vi "Measure Harmonic Distortion.vi"(9 "Auto cal (F)?":bool, 11 "State":T1) -> (0 "error out":errorcluster)   [LabVIEW 2015]
uses:
  Utility VIs/Type Defs/Speaker ring.ctl
  Utility VIs/Buttons/KCheckmarkBoolean 2.ctl
  Cochlear Function Test Suite/LV Source/CFTS Main Panel SubVIs/CFTS-Experiment State.ctl
  Type Defs/ACal-In Ear Parameters.ctl
  Type Defs/Cal Stimulus.ctl
  Type Defs/ACal-Multiband Parameters.ctl
  Utility VIs/Conversion VIs/Create Waveform Cluster (2D).vi
  Utility VIs/Math VIs/FFT x(t) to dB,Degrees (2D).vi
  Instance           1 24Saved   Calibrate In Ear .vi
  Utility VIs/File IO VIs/Configuration File Wrapper VIs/Config-Read Key (Boolean).vi
panel:
  in  "Weighted":bool
  out "Auto Message":string="Auto calibrating!"
  in  "Speaker":T2
  in  "mic gain":dbl caption="Probe Mic Gain (dB)"
  in  "Stimulus":T3={"Min Freq (Hz)"=1000.0, "Max Freq (Hz)"=50000.0, "Freq Step (Hz)"=50.0, "Waveform"=0, "Attenuation (dB)"=30.0, "Sample Rate (Hz)"=100000.0} {"Waveform" items=["Chirp", "Weighted"]}
  out "Stimulus graph":cluster{i32, dbl, dbl[]}(graph)={0, 0.01, []}
  in  "Averages":i32=128
  in  "Return":bool
  in  "START":bool
  in  "STOP":bool
  in  "result":cluster{"Path":path, "error ":errorcluster}
  in  "Plot Max SPL":T4=TRUE
  out "ASTF":cluster{"Frequency":dbl[], "Frequency":dbl[]}[](graph)
  in  "Last N":bool
  in  "Show all":bool
  in  "Load":bool
  in  "Clear":bool
  out "Path":path
  out "Acquired":i32=256
  out "ASTF phase":cluster{"Frequency":dbl[], "Frequency":dbl[]}[](graph)
  out "Mic phase graph":cluster{"offset":dbl, "dx":dbl, "Y":dbl[][]}(graph)
  out "Mic mag":cluster{"offset":dbl, "dx":dbl, "Y":dbl[][]}(graph)
  out "Mic signals":cluster{"offset":dbl, "dx":dbl, "Y":dbl[][]}(graph)
  # "Raw Data"
  # "Acoustic System Transfer Function"
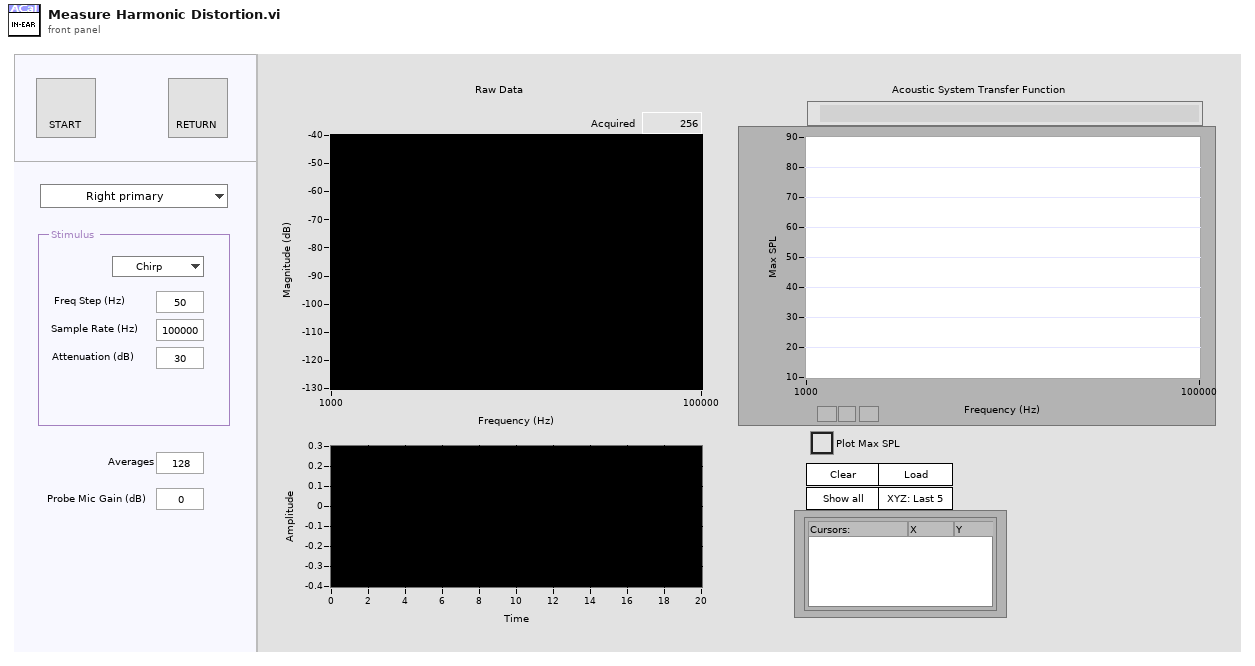
[diagram p1: front panel]
types:
  T1 = typedef "CFTS-Experiment State.ctl" = cluster{"Experimenter":string, "Number":u32, "Right":string, "Left":string, "Data Folder":path, "State File":path, "Version Info":string, "End Exposure Time":dbl, "Exposure Duration":string, "Run #":cluster{"CAP":i16, "ABR":i16, "DP":i16, "VsEP":i16, "MeasSeq":i16, "SubSeq":i16, "SFOAE":i16}}
  T2 = typedef "Speaker ring.ctl" = enum16{"Right primary", "Right secondary", "Left primary", "Left secondary"}
  T3 = cluster{"Min Freq (Hz)":dbl, "Max Freq (Hz)":dbl, "Freq Step (Hz)":dbl, "Waveform":u16, "Attenuation (dB)":dbl, "Sample Rate (Hz)":dbl}
  T4 = typedef "KCheckmarkBoolean 2.ctl" = bool
  T5 = typedef "ACal-In Ear Parameters.ctl" = cluster{"Speaker":T2, "Stimulus":T6, "Averages":i32, "Left gain":dbl, "Right gain":dbl, "plot max":bool, "smooth override":bool, "Weighted":T7}
  T6 = typedef "Cal Stimulus.ctl" = cluster{"Min Freq (Hz)":dbl, "Max Freq (Hz)":dbl, "Freq Step (Hz)":dbl, "Waveform":enum16{"Chirp", "Weighted"}, "Attenuation (dB)":dbl, "Sample Rate (Hz)":dbl}
  T7 = typedef "ACal-Multiband Parameters.ctl" = cluster{"Folder":path, "Fmin":dbl, "Fmax":dbl, "Max range":dbl, "WF":u16}
  T8 = typedef "Cal-Smoothing Parameters.ctl" = cluster{"Method":enum16{"None", "Moving average", "Loess"}, "MA":cluster{"Iterations":i32, "Length":i32}, "Loess":cluster{"Length":i32, "Type":enum16{"Linear", "Quadratic"}, "Robust":bool}}
  T9 = cluster{"new file path":path, "error out":errorcluster}
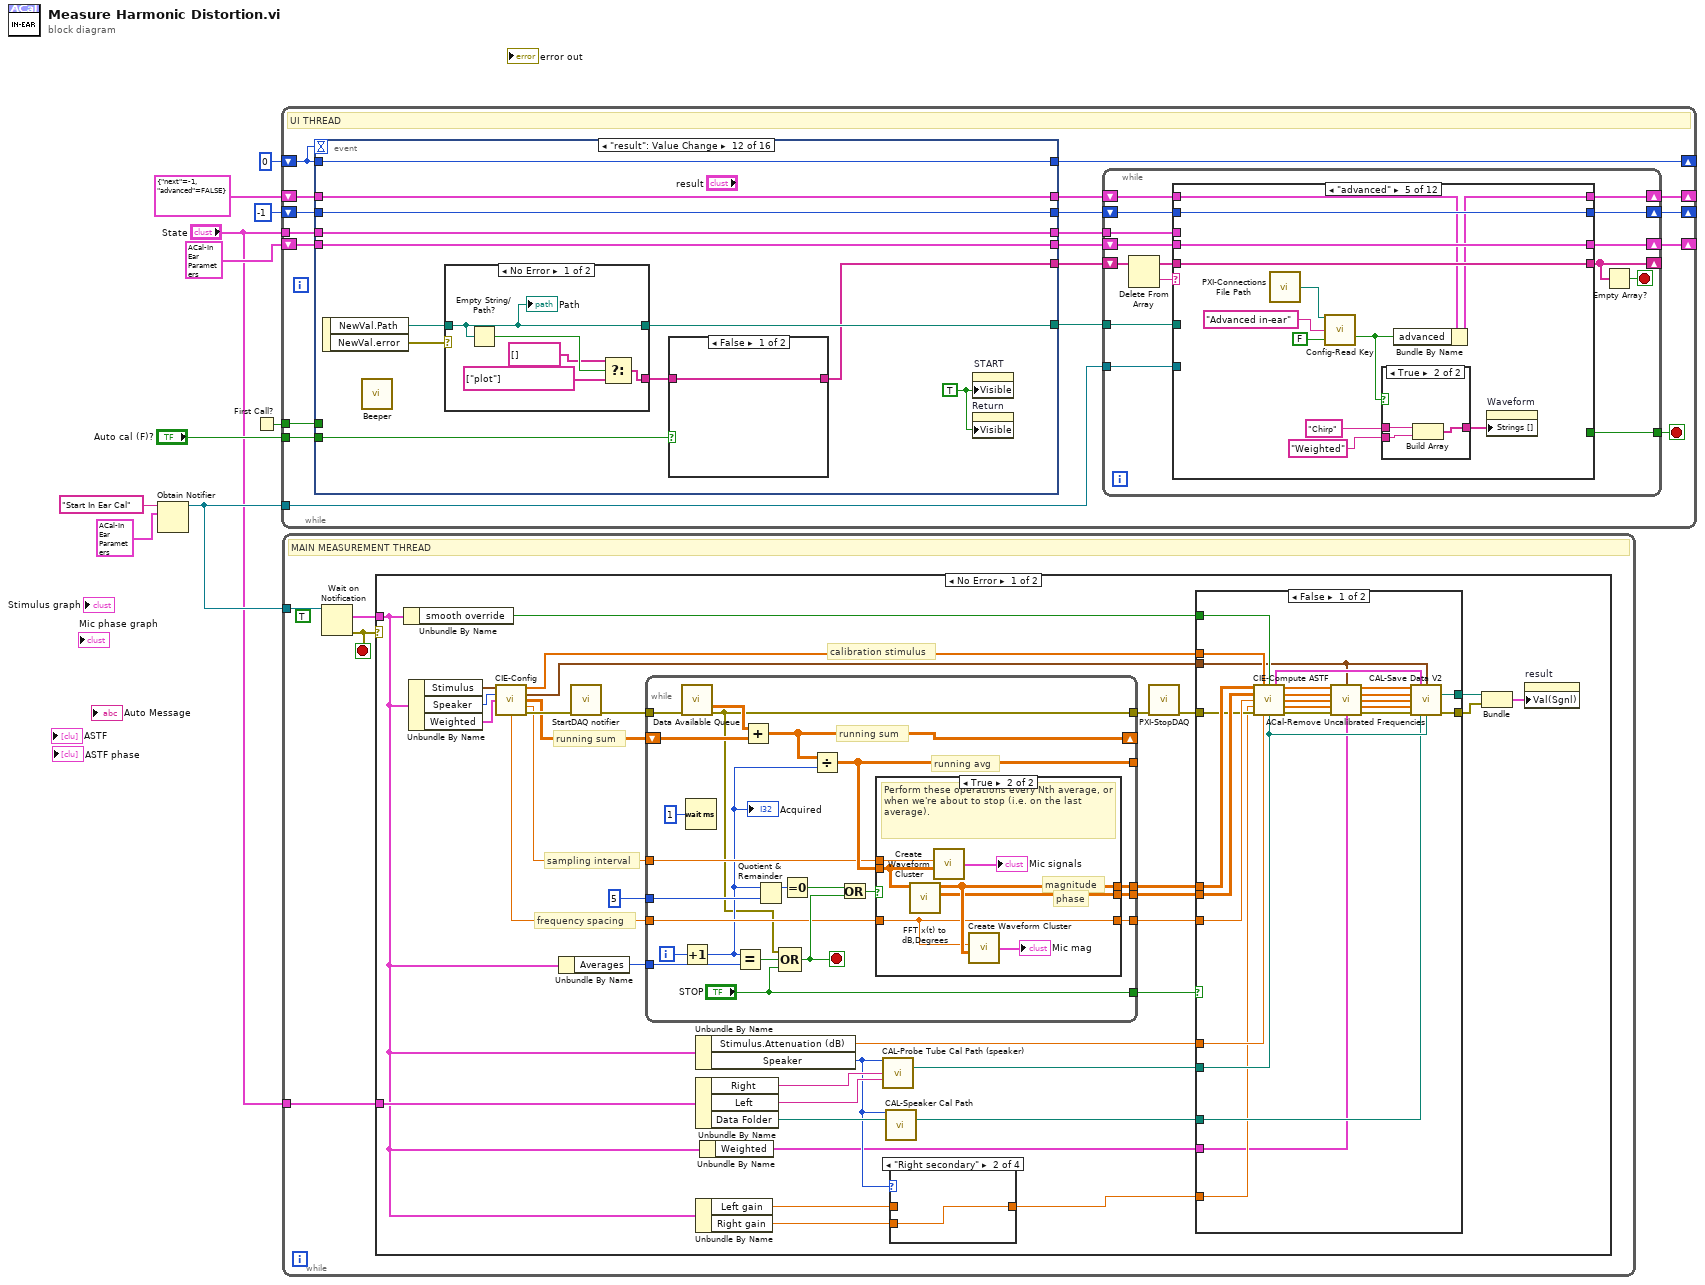
[diagram p0: block diagram]
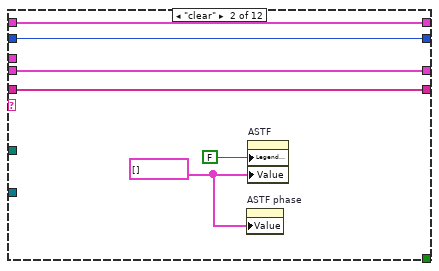
[diagram p9: hidden frame]
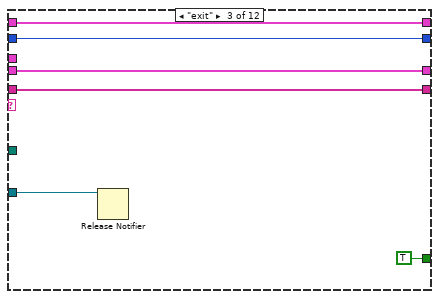
[diagram p10: hidden frame]
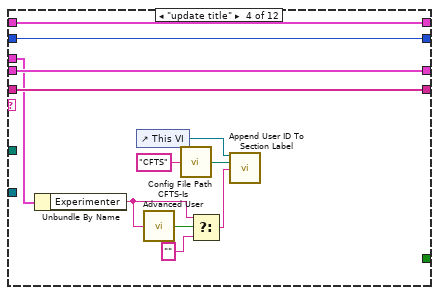
[diagram p11: hidden frame]
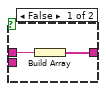
[diagram p12: hidden frame]
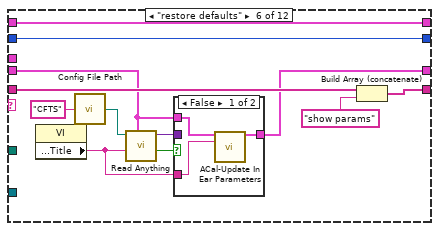
[diagram p13: hidden frame]
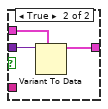
[diagram p14: hidden frame]
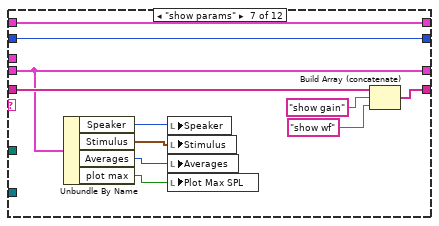
[diagram p15: hidden frame]
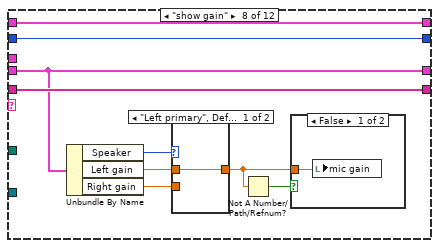
[diagram p16: hidden frame]
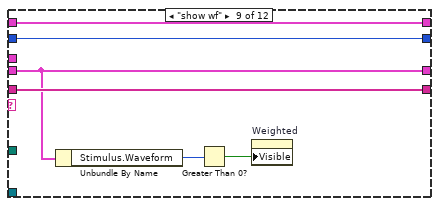
[diagram p19: hidden frame]
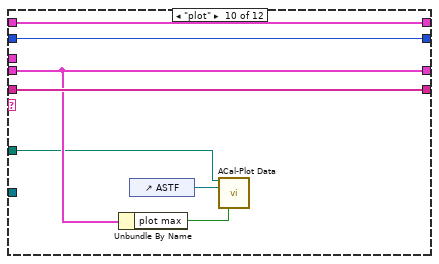
[diagram p20: hidden frame]
diagram:
  n1 = Obtain Notifier(name (unnamed)="Start In Ear Cal", notification data type=T5 {"Speaker"=enum."Right primary", "Stimulus"={"Min Freq (Hz)"=50.0, "Max Freq (Hz)"=50000.0, "Freq Step (Hz)"=50.0, "Waveform"=enum."Chirp", "Attenuation (dB)"=20.0, "Sample Rate (Hz)"=100000.0}, "Averages"=512, "Left gain"=40.0, "Right gain"=40.0, "plot max"=TRUE, "smooth override"=FALSE, "Weighted"={"Folder"=path "", "Fmin"=0.0, "Fmax"=0.0, "Max range"=0.0, "WF"=0}} ("Params")) -> (notifier out=w10:refnum<notifier>)  [unwired: 2 in, 2 out]
  n2 = First Call?() -> (First Call?: T/F=w1:bool)
  n3 = while {
    tunnel: w10 -> [w17]
    shift-right: [w26] -> _
    shift-left: 0 -> [w27]
    tunnel: "Auto cal (F)?" -> [w29]
    shift-right: [w20] -> _
    shift-left: -1 -> [w28]
    tunnel: "State" -> [w25]
    shift-right: [w21] -> _
    shift-left: T5 {"Speaker"=enum."Right primary", "Stimulus"={"Min Freq (Hz)"=50.0, "Max Freq (Hz)"=50000.0, "Freq Step (Hz)"=50.0, "Waveform"=enum."Chirp", "Attenuation (dB)"=20.0, "Sample Rate (Hz)"=100000.0}, "Averages"=512, "Left gain"=40.0, "Right gain"=40.0, "plot max"=TRUE, "smooth override"=FALSE, "Weighted"={"Folder"=path "C:/Data", "Fmin"=3000.0, "Fmax"=45000.0, "Max range"=25.0, "WF"=0}} ("Params") -> [w24]
    shift-right: [w12] -> _
    shift-left: cluster{"next":i32, "advanced":bool} {"next"=-1, "advanced"=FALSE} -> [w14]
    tunnel: w1 -> [w11]
    stop <- w18 stop-if-true
    # "UI THREAD"
    n4 = event shown="[11] \"result\": Value Change" {
      selector: _ -> [_ _ _ _ _ _ _ _ _ _ _ _ _ _ _ _]
      dyn-events: _ -> [_ _ _ _ _ _ _ _ _ _ _ _ _ _ _ _]
      timeout: w27 -> [_ _ _ _ _ _ _ _ _ _ _ _ _ _ _ _]
      tunnel: w29 -> [w184 _ _ _ _ _ _ _ _ _ _ w307 _ _ _ _]
      tunnel: w28 -> [w185 w202 w211 w233 w239 w247 w250 w263 w265 w278 w291 w315 w331 w338 w353 w363]
      tunnel: [w185 w202 w211 w233 w239 w247 w250 w263 w265 w278 w291 w315 w331 w338 w353 w363] -> w23
      tunnel: w27 -> [_ w201 w210 w232 w238 w246 w255 w262 w270 w277 w290 w314 w330 w337 w351 w361]
      tunnel: [-1 w201 w210 w232 w238 w246 w255 w262 w270 w277 w290 w314 w330 w337 w351 w361] -> w26
      tunnel: w25 -> [w180 w198 w205 w229 w237 w241 w253 w261 w268 w273 w288 w312 w327 w335 w350 w360]
      tunnel: w24 -> [w182 w200 w208 w231 w236 w245 w254 w259 w269 w275 w289 w313 w329 w336 w349 w359]
      tunnel: [w182 w200 w207 w231 w236 w243 w252 w257 w267 w274 w287 w313 w329 w336 w349 w359] -> w22
      tunnel: [w179 string[] ["exit"] w206 string[] ["exit"] string[] ["start"] string[] ["show gain"] string[] ["show wf"] _ _ _ _ w305 string[] ["clear"] w333 _ _] -> w19
      tunnel: [w180 w198 w205 w229 w237 w241 w253 w261 w268 w273 w288 w312 w327 w335 w350 w360] -> w16
      tunnel: [_ _ _ _ _ _ _ _ _ _ _ w310 _ w334 _ _] -> w15
      tunnel: w14 -> [w177 w197 w204 w228 w235 w240 w249 w260 w264 w271 w285 w309 w326 w332 w347 w356]
      tunnel: [w177 w197 w204 w228 w235 w240 w249 w260 w264 w271 w285 w309 w326 w332 w347 w356] -> w13
      tunnel: w11 -> [w175 _ _ _ _ _ _ _ _ _ _ _ _ _ _ _]
      event Timeout {
        w191 = TRUE ("Visible")
        n5 = event-data() -> ()  [unwired: 1 in, 1 out]
        n6 = case shown="False" w184 {
          tunnel: [w193 string[] ["next", "clear"]] -> w181
          tunnel: w175 -> [w195 _]
          frame False {
            n7 = Select(t=string[] ["clear"], s=w195, f=string[] []) -> (s? t:f=w193:string[])
          }
          frame True {
          }
        }
        n8 = property on="Auto Message" class="Str"("Visible"=w184, "Blinking"=w184) -> ()  [unwired: 2 in, 2 out]
        n9 = Unbundle By Name(w180) -> ("Experimenter"=w190:string)
        n10 = property on="Weighted" class="Bool"("Visible"=FALSE) -> ()  [unwired: 2 in, 2 out]
        n11 = Concatenate Strings(w190, ": Last 5" ("string")) -> (w188:string)
        n12 = property on="START" class="Bool"("Visible"=w191) -> ()  [unwired: 2 in, 2 out]
        n13 = property on="Return" class="Bool"("Visible"=w191) -> ()  [unwired: 2 in, 2 out]
        n14 = Initialize Array(w188, 4 ("dimension size")) -> (w186:string[])
        n15 = property on="Last N" class="Bool"("Strings [4]"=w186) -> ()  [unwired: 2 in, 2 out]
        n16 = Build Array (concatenate)(w181, string[] ["restore defaults", "advanced", "update title"]) -> (w179:string[])
      }
      event Panel Close? {
        n17 = event-data() -> ()  [unwired: 1 in, 1 out]
        n18 = event-data("Discard?"=TRUE) -> ()  [unwired: 1 in, 1 out]
      }
      event Menu Selection (User) {
        n19 = event-data() -> ("ItemTag"=w209:string)  [unwired: 1 in]
        n20 = case shown="\"mmFileSave\"" w209 {
          tunnel: w208 -> [w212 w214 w217 w223 w226]
          tunnel: [w212 w214 w217 w223 w224] -> w207
          tunnel: [_ string[] ["restore defaults"] _ string[] ["exit"] _] -> w206
          frame "", Default {
          }
          frame "mmFileRestore" {
          }
          frame "mmFileSave" {
            n21 = property class="VI"() -> ("Front Panel.Title"=w216:string)  [unwired: 2 in, 2 out]
            n22 = call "Config File Path.vi"("AppName"="CFTS") -> ("Default config file name"=w218:path)
            n23 = call "Write Anything.vi"("Section Name (Name of \"Anything\")"=w216, "Anything"=w217, "Path (dialog)"=w218) -> ("Error Out"=w215:errorcluster)  [unwired: 7 in, 1 out]
            n24 = case shown="Error" w215 {
              selector: w215 -> [_ w221]
              frame No Error {
                n25 = One Button Dialog(message="Defaults saved.") -> ()  [unwired: 1 in, 1 out]
              }
              frame Error {
                n26 = call "Error Handler.vi"("error in (no error)"=w221) -> ()  [unwired: 13 in, 2 out]
              }
            }
          }
          frame "mmFileExit" {
          }
          frame "mmEditOptions" {
            n27 = Unbundle By Name(w226) -> ("smooth override"=w227:bool)
            n28 = call "CIE-Options Dialog.vi"("Override smoothing"=w227) -> ("Override Out"=w225:bool)  [unwired: 13 in, 1 out]
            n29 = Bundle By Name(cluster=w226, "smooth override"=w225) -> (w224:T5)
          }
        }
      }
      event "Return": Value Change {
        n30 = event-data() -> ()  [unwired: 1 in, 1 out]
      }
      event "START": Value Change {
        n31 = event-data() -> ()  [unwired: 1 in, 1 out]
      }
      event Value Change {
        n32 = event-data() -> ("NewVal"=w242:T2)  [unwired: 1 in]
        n33 = Bundle By Name(cluster=w245, "Speaker"=w242) -> (w243:T5)
      }
      event "Stimulus": Value Change {
        n34 = event-data() -> ()  [unwired: 1 in, 1 out]
        n35 = Bundle By Name(cluster=w254, "Stimulus"="Stimulus") -> (w252:T5)
      }
      event "Weighted": Value Change {
        n36 = event-data() -> ()  [unwired: 1 in, 1 out]
        n37 = Unbundle By Name(w259) -> ("Weighted"=w258:T7)
        n38 = call "ACal-Multiband Dialog.vi"("Cluster In"=w258) -> ("Cluster out"=w256:T7)  [unwired: 13 in, 1 out]
        n39 = Bundle By Name(cluster=w259, "Weighted"=w256) -> (w257:T5)
      }
      event "Averages": Value Change {
        n40 = event-data() -> ()  [unwired: 1 in, 1 out]
        n41 = Bundle By Name(cluster=w269, "Averages"="Averages") -> (w267:T5)
      }
      event "mic gain": Value Change {
        n42 = event-data() -> ()  [unwired: 1 in, 1 out]
        n43 = Unbundle By Name(w275) -> ("Speaker"=w276:T2)
        n44 = case shown="\"Right primary\", \"Right secondary\"" w276 {
          tunnel: w275 -> [w281 w284]
          tunnel: [w280 w283] -> w274
          tunnel: "mic gain" -> [w279 w282]
          frame "Left primary", Default {
            n45 = Bundle By Name(cluster=w281, "Left gain"=w279) -> (w280:T5)
          }
          frame "Right primary", "Right secondary" {
            n46 = Bundle By Name(cluster=w284, "Right gain"=w282) -> (w283:T5)
          }
        }
      }
      event Value Change {
        # "Clear the plot because the scaling is no longer consistent with the option. We haven't retained a list of displayed data files, so we can't restore them with the proper scaling. The best we can do (without more serious revision) is to reload the last saved calibration file."
        n47 = event-data() -> ("NewVal"=w296:T4)  [unwired: 1 in]
        n48 = control-ref of="ASTF"() -> (w294:refnum<vi>)
        n49 = property class="XYGraph (strict)"(reference=w294, "Value"=cluster{"Frequency":dbl[], "Frequency":dbl[]}[] []) -> (reference out=w292:refnum<vi>, error out=w295:errorcluster)  [unwired: 1 in]
        n50 = Bundle By Name(cluster=w289, "plot max"="Plot Max SPL") -> (w287:T5)
        n51 = local read "Path"() -> (w298:path)
        n52 = call "FileIO-File or Folder Exists.vi"("error in (no error)"=w295, "path"=w298) -> ("Directory?"=w299:bool, "dup path"=w297:path)  [unwired: 6 in, 2 out]
        n53 = case shown="True" w299 {
          tunnel: w292 -> [_ w302]
          tunnel: w296 -> [_ w300]
          tunnel: w297 -> [_ w303]
          frame False {
          }
          frame True {
            n54 = call "ACal-Plot Data.vi"("Path"=w303, "Mag graph"=w302, "Plot max"=w300) -> ("error out"=w301:errorcluster)  [unwired: 11 in, 1 out]
            n55 = call <vilib>:"Simple Error Handler.vi"("error in (no error)"=w301) -> ()  [unwired: 4 in, 5 out]
          }
        }
      }
      event "result": Value Change {
        w308 = TRUE
        n56 = event-data() -> ("NewVal.Path"=w311:path, "NewVal.error"=w304:errorcluster)  [unwired: 1 in]
        n57 = call "Beeper.vi"() -> ()  [unwired: 5 in, 1 out]
        n58 = case shown="No Error" w304 {
          selector: w304 -> [_ w325]
          tunnel: w311 -> [w324 _]
          tunnel: [w324 _] -> w310
          tunnel: [w321 _] -> w306
          frame No Error {
            n59 = Empty String/Path?(string/path=w324) -> (empty?=w323:bool)
            n60 = Select(t=string[] [], s=w323, f=string[] ["plot"]) -> (s? t:f=w321:string[])
            "Path" <- w324
          }
          frame Error {
            n61 = call "Error Handler.vi"("error in (no error)"=w325) -> ()  [unwired: 13 in, 2 out]
          }
        }
        n62 = case shown="False" w307 {
          tunnel: w306 -> [w316 w319]
          tunnel: [w316 w318] -> w305
          frame False {
          }
          frame True {
            n63 = Build Array (concatenate)("next", w319) -> (w318:string[])
          }
        }
        n64 = property on="START" class="Bool"("Visible"=w308) -> ()  [unwired: 2 in, 2 out]
        n65 = property on="Return" class="Bool"("Visible"=w308) -> ()  [unwired: 2 in, 2 out]
      }
      event "Clear": Value Change {
        n66 = event-data() -> ()  [unwired: 1 in, 1 out]
      }
      event "Load": Value Change {
        n67 = event-data() -> ()  [unwired: 1 in, 1 out]
        n68 = Unbundle By Name(w335) -> ("Data Folder"=w339:path)
        n69 = call "File Dialog"("start path"=w339, "pattern (all files)"="*.calib", "pattern label"="Calibration files") -> ("selected path"=w344:path, "cancelled"=w343:bool, "error out"=w342:errorcluster)  [unwired: 9 in, 1 out]
        n70 = case shown="False" w343 {
          tunnel: w344 -> [w346 _]
          tunnel: w342 -> [_ _]
          tunnel: [w346 _] -> w334
          tunnel: [string[] ["plot"] _] -> w333
          frame False {
          }
          frame True {
          }
        }
      }
      event "Show all": Value Change {
        n71 = event-data() -> ()  [unwired: 1 in, 1 out]
        n72 = Unbundle By Name(w349) -> ("plot max"=w348:bool)
        n73 = Unbundle By Name(w350) -> ("Data Folder"=w354:path)
        n74 = control-ref of="ASTF"() -> (w352:refnum<vi>)
        n75 = call "CAL-Show all.vi"("Path"=w354, "Mag graph"=w352, "Plot Max SPL"=w348) -> ("error out"=w355:errorcluster)  [unwired: 11 in, 1 out]
        n76 = call "Error Handler.vi"("error in (no error)"=w355) -> ()  [unwired: 13 in, 2 out]
      }
      event "Last N": Value Change {
        n77 = event-data() -> ()  [unwired: 1 in, 1 out]
        n78 = Unbundle By Name(w359) -> ("Speaker"=w357:T2, "plot max"=w358:bool)
        n79 = control-ref of="ASTF"() -> (w362:refnum<vi>)
        n80 = call "CAL-Show Last N.vi"("Expt State"=w360, "Mag graph"=w362, "Speaker"=w357, "Plot Max SPL"=w358) -> ("error out"=w364:errorcluster)  [unwired: 11 in]
        n81 = call <vilib>:"Simple Error Handler.vi"("error in (no error)"=w364) -> ()  [unwired: 4 in, 5 out]
      }
    }
    n82 = while {
      shift-right: [w42] -> w21
      shift-left: w22 -> [w43]
      shift-right: [w41] -> w20
      shift-left: w23 -> [w44]
      shift-right: [w37] -> _
      shift-left: w19 -> [w39]
      tunnel: w17 -> [w35]
      tunnel: [w34] -> w18
      tunnel: w16 -> [w33]
      tunnel: w15 -> [w32]
      shift-right: [w31] -> w12
      shift-left: w13 -> [w30]
      stop <- w36 stop-if-true
      n83 = Delete From Array(array=w39) -> (deleted portion=w38:string, array with subset deleted=w40:string[])  [unwired: 2 in]
      n84 = case shown="\"advanced\"" w38 {
        tunnel: w44 -> [w48 w54 w60 w72 w84 w101 w118 w127 w136 w143 w149 w162]
        tunnel: [w48 w54 w60 w72 w84 w101 w118 w127 w136 w143 w149 w162] -> w41
        tunnel: w43 -> [w47 w53 w59 w71 w83 w96 w116 w125 w133 w141 w144 w155]
        tunnel: [w47 w53 w59 w71 w83 w95 w116 w125 w133 w141 w144 w154] -> w42
        tunnel: w40 -> [w46 w52 w58 w70 w82 w100 w117 w126 w135 w142 w145 w153]
        tunnel: [w46 w52 w58 w70 w82 w94 w111 w126 w135 w142 w145 w150] -> w37
        tunnel: w35 -> [_ _ w57 _ _ _ _ _ _ _ w146 _]
        tunnel: [_ _ TRUE _ _ _ _ _ _ _ _ w158] -> w34
        tunnel: w33 -> [_ _ _ w63 _ _ _ _ _ _ _ _]
        tunnel: w32 -> [_ _ _ _ _ _ _ _ _ w138 _ _]
        tunnel: [w45 w49 w55 w61 w77 w90 w109 w119 w134 w137 w148 w151] -> w31
        tunnel: w30 -> [w45 w49 w55 w61 w78 w90 w109 w119 w134 w137 w148 w152]
        frame "", Default {
        }
        frame "clear" {
          w51 = cluster{"Frequency":dbl[], "Frequency":dbl[]}[] [] ("ASTF mag")
          n85 = property on="ASTF phase" class="XYGraph (strict)"("Value"=w51) -> ()  [unwired: 2 in, 2 out]
          n86 = property on="ASTF" class="XYGraph (strict)"("Legend Visible"=FALSE ("Legend:Visible"), "Value"=w51) -> ()  [unwired: 2 in, 2 out]
        }
        frame "exit" {
          n87 = Release Notifier(notifier=w57) -> ()  [unwired: 2 in, 3 out]
        }
        frame "update title" {
          n88 = Unbundle By Name(w63) -> ("Experimenter"=w62:string)
          n89 = control-ref of="This VI"() -> (w64:refnum<vi>)
          n90 = call "CFTS-Is Advanced User.vi"("Experimenter"=w62) -> ("Advanced user"=w67:bool)
          n91 = call "Config File Path.vi"("AppName"="CFTS") -> ("Default config file name"=w65:path)
          n92 = Select(t=w62, s=w67, f="") -> (s? t:f=w69:string)
          n93 = call "Append User ID To Section Label.vi"("VI reference"=w64, "Path (dialog)"=w65, "User"=w69) -> ()  [unwired: 9 in, 4 out]
        }
        frame "advanced" {
          n94 = call "PXI-Connections File Path.vi"() -> ("Path"=w79:path)  [unwired: 1 in]
          n95 = call-poly "Config-Read Key.vi"("configuration file path"=w79, "key"="Advanced in-ear", "default"=FALSE) -> ("value"=w76:bool)  [unwired: 9 in, 3 out]
          n96 = case shown="True" w76 {
            tunnel: "Chirp" ("key") -> [w86 w89]
            tunnel: "Weighted" ("key") -> [_ w88]
            tunnel: [w85 w87] -> w73
            frame False {
              n97 = Build Array(w86) -> (w85:string[])
            }
            frame True {
              n98 = Build Array(w89, w88) -> (w87:string[])
            }
          }
          n99 = Bundle By Name(cluster=w78, "advanced"=w76) -> (w77:cluster{"next":i32, "advanced":bool})
          n100 = property on="Waveform" class="Ring (strict)"("Strings []"=w73) -> ()  [unwired: 2 in, 2 out]
        }
        frame "restore defaults" {
          n101 = property class="VI"() -> ("Front Panel.Title"=w92:string)  [unwired: 2 in, 2 out]
          n102 = call "Config File Path.vi"("AppName"="CFTS") -> ("Default config file name"=w91:path)
          n103 = call "Read Anything.vi"("Type of Anything"=w96, "Section Name (Name of \"Type of Anything\")"=w92, "Path (dialog)"=w91) -> ("Found?"=w98:bool, "Anything"=w97:variant)  [unwired: 6 in, 1 out]
          n104 = case shown="False" w98 {
            tunnel: w97 -> [_ w107]
            tunnel: w96 -> [w104 w106]
            tunnel: [w103 w105] -> w95
            tunnel: w92 -> [w102 _]
            frame False {
              n105 = call "ACal-Update In Ear Parameters.vi"("Params in"=w104, "Section"=w102) -> ("Params out"=w103:T5)  [unwired: 13 in]
            }
            frame True {
              n106 = Variant To Data(type=w106, Variant=w107) -> (data=w105:T5)  [unwired: 1 in, 1 out]
            }
          }
          n107 = Build Array (concatenate)(w100, "show params") -> (w94:string[])
        }
        frame "show params" {
          n108 = Unbundle By Name(w116) -> ("Speaker"=w115:T2, "Stimulus"=w114:T6, "Averages"=w113:i32, "plot max"=w112:bool)
          n109 = local write "Speaker"(w115) -> ()
          n110 = local write "Stimulus"(w114) -> ()
          n111 = local write "Averages"(w113) -> ()
          n112 = local write "Plot Max SPL"(w112) -> ()
          n113 = Build Array (concatenate)(w117, "show gain", "show wf") -> (w111:string[])
        }
        frame "show gain" {
          n114 = Unbundle By Name(w125) -> ("Speaker"=w122:T2, "Left gain"=w121:dbl, "Right gain"=w120:dbl)
          n115 = case shown="\"Left primary\", Default" w122 {
            tunnel: w121 -> [w129 _]
            tunnel: w120 -> [_ w130]
            tunnel: [w129 w130] -> w124
            frame "Left primary", Default {
            }
            frame "Right primary", "Right secondary" {
            }
          }
          n116 = Not A Number/Path/Refnum?(number/path/refnum=w124) -> (NaN/Path/Refnum?=w123:bool)
          n117 = case shown="False" w123 {
            tunnel: w124 -> [w128 _]
            frame False {
              n118 = local write "mic gain"(w128) -> ()
            }
            frame True {
            }
          }
        }
        frame "show wf" {
          n119 = Unbundle By Name(w133) -> ("Stimulus.Waveform"=w132:enum16{"Chirp", "Weighted"})
          n120 = Greater Than 0?(x=w132) -> (x > 0?=w131:bool)
          n121 = property on="Weighted" class="Bool"("Visible"=w131) -> ()  [unwired: 2 in, 2 out]
        }
        frame "plot" {
          n122 = Unbundle By Name(w141) -> ("plot max"=w140:bool)
          n123 = control-ref of="ASTF"() -> (w139:refnum<vi>)
          n124 = call "ACal-Plot Data.vi"("Path"=w138, "Mag graph"=w139, "Plot max"=w140) -> ()  [unwired: 11 in, 2 out]
        }
        frame "start" {
          w147 = FALSE
          n125 = Send Notification(notification=w144, notifier=w146) -> ()  [unwired: 1 in, 2 out]
          n126 = property on="Return" class="Bool"("Visible"=w147) -> ()  [unwired: 2 in, 2 out]
          n127 = property on="START" class="Bool"("Visible"=w147) -> ()  [unwired: 2 in, 2 out]
        }
        frame "next" {
          w157 = T2[] [enum."Right primary", enum."Right secondary", enum."Left primary", enum."Left secondary"] items=["Right primary", "Right secondary", "Left primary", "Left secondary"]
          n128 = Unbundle By Name(w152) -> ("next"=w161:i32)
          n129 = Array Size(array=w157) -> (size(s)=w160:i32)
          n130 = Increment(x=w161) -> (x+1=w156:i32)
          n131 = Less?(x=w156, y=w160) -> (x < y?=w159:bool)
          n132 = case shown="True" w159 {
            tunnel: [TRUE _] -> w158
            tunnel: w157 -> [_ w174]
            tunnel: w156 -> [_ w169]
            tunnel: w155 -> [w165 w173]
            tunnel: [w165 w171] -> w154
            tunnel: [w164 string[] ["start"]] -> w150
            tunnel: w153 -> [w164 _]
            tunnel: w152 -> [w163 w170]
            tunnel: [w163 w168] -> w151
            frame False {
            }
            frame True {
              n133 = Index Array(array=w174, index=w169) -> (element=w172:T2)
              n134 = Bundle By Name(cluster=w173, "Speaker"=w172) -> (w171:T5)
              n135 = local write "Speaker"(w172) -> ()
              n136 = Bundle By Name(cluster=w170, "next"=w169) -> (w168:cluster{"next":i32, "advanced":bool})
            }
          }
        }
      }
      n137 = Empty Array?(array=w37) -> (empty?=w36:bool)
    }
  }
  n138 = while {
    tunnel: w10 -> [w368]
    tunnel: "State" -> [w366]
    stop <- w367 stop-if-true
    (unwired) TRUE
    # "MAIN MEASUREMENT THREAD"
    n139 = Wait on Notification(notifier=w368) -> (notification=w365:T5, error out=w367:errorcluster)  [unwired: 3 in, 2 out]
    n140 = case shown="No Error" w367 {
      tunnel: w366 -> [w385 _]
      tunnel: w365 -> [w370 _]
      frame No Error {
        # "calibration stimulus"
        # "frequency spacing"
        # "sampling interval"
        # "running sum"
        n141 = Unbundle By Name(w370) -> ("smooth override"=w381:bool)
        n142 = Unbundle By Name(w370) -> ("Stimulus"=w384:T6, "Speaker"=w383:T2, "Weighted"=w371:T7)
        n143 = call "CIE-Config.vi"("Cal Stimulus"=w384, "Speaker"=w383, "Weighted"=w371) -> ("Stimulus"=w396:dbl[], "Cal Spec Out"=w387:T6, "Mic Avg"=w402:dbl[][], "dt (ms)"=w400:dbl, "df (Hz)"=w401:dbl, "error out"=w403:errorcluster)  [unwired: 6 in, 1 out]
        n144 = Unbundle By Name(w370) -> ("Averages"=w382:i32)
        n145 = call "StartDAQ notifier.vi"("error in (no error)"=w403) -> ("error out"=w395:errorcluster)  [unwired: 6 in]
        n146 = while {
          tunnel: w395 -> [w455]
          tunnel: [w435] -> w394
          tunnel: w382 -> [w452]
          shift-right: [w450] -> _
          shift-left: w402 -> [w451]
          tunnel: [w449] -> _
          tunnel: 5 -> [w448]
          tunnel: w401 -> [w443]
          tunnel: [w442] -> w399
          tunnel: [w441] -> w398
          tunnel: w400 -> [w440]
          tunnel: [w439] -> w397
          tunnel: ["STOP"] -> w379
          i -> [w454]
          stop <- w444 stop-if-true
          # "running avg"
          # "running sum"
          n147 = call "Data Available Queue.vi"("error in (no error)"=w455) -> ("AI Waveforms"=w437:dbl[][], "error out"=w435:errorcluster)  [unwired: 10 in, 3 out]
          n148 = Increment(x=w454) -> (x+1=w438:i32)
          "Acquired" <- w438
          n149 = Wait (ms)(milliseconds to wait=u32 1) -> ()  [unwired: 1 out]
          n150 = Equal?(x=w438, y=w452) -> (x = y?=w453:bool)
          n151 = Add(x=w437, y=w451) -> (x+y=w450:dbl[][])
          n152 = Quotient & Remainder(x=w438, y=w448) -> (x-y*floor(x/y)=w447:i32)  [unwired: 1 out]
          n153 = Compound Arithmetic op=OR(w435, w453, "STOP") -> (w444:bool)
          n154 = Equal To 0?(x=w447) -> (x = 0?=w445:bool)
          n155 = Divide(x=w450, y=w438) -> (x/y=w449:dbl[][])
          n156 = Or(x=w445, y=w444) -> (x .or. y?=w446:bool)
          n157 = case shown="True" w446 {
            tunnel: w449 -> [_ w459]
            tunnel: w443 -> [_ w456]
            tunnel: [_ w461] -> w442
            tunnel: [_ w460] -> w441
            tunnel: w440 -> [_ w458]
            tunnel: [_ w456] -> w439
            frame False {
            }
            frame True {
              # "phase"
              # "magnitude"
              # "Perform these operations every Nth average, or when we're about to stop (i.e. on the last average)."
              n158 = call-poly "FFT x(t) to dB,Degrees.vi"("X(t)"=w459) -> ("+Freq Phase of FFT (degrees)"=w460:dbl[][], "+Freq. Mag of FFT (dB rms)"=w461:dbl[][])  [unwired: 9 in]
              n159 = call-poly "Create Waveform Cluster.vi"("dx"=w458, "Array"=w459) -> ("waveform cluster"=→"Mic signals":cluster{"offset":dbl, "dx":dbl, "Y":dbl[][]})  [unwired: 3 in]
              n160 = call-poly "Create Waveform Cluster.vi"("dx"=w456, "Array"=w461) -> ("waveform cluster"=→"Mic mag":cluster{"offset":dbl, "dx":dbl, "Y":dbl[][]})  [unwired: 3 in]
            }
          }
        }
        n161 = Unbundle By Name(w370) -> ("Stimulus.Attenuation (dB)"=w380:dbl, "Speaker"=w378:T2)
        n162 = Unbundle By Name(w385) -> ("Right"=w392:string, "Left"=w391:string, "Data Folder"=w390:path)
        n163 = Unbundle By Name(w370) -> ("Left gain"=w377:dbl, "Right gain"=w375:dbl)
        n164 = Unbundle By Name(w370) -> ("Weighted"=w369:T7)
        n165 = call "CAL-Probe Tube Cal Path (speaker).vi"("Speaker"=w378, "Right"=w392, "Left"=w391) -> ("Probe Tube Cal Path"=w389:path)  [unwired: 11 in, 1 out]
        n166 = call "CAL-Speaker Cal Path.vi"("Speaker"=w378, "Data Folder"=w390) -> ("Cal Path"=w386:path)  [unwired: 12 in, 1 out]
        n167 = case shown="\"Right secondary\"" w378 {
          tunnel: w377 -> [_ _ w406 w407]
          tunnel: [w404 w405 w406 w407] -> w376
          tunnel: w375 -> [w404 w405 _ _]
          frame "Right primary", Default {
          }
          frame "Right secondary" {
          }
          frame "Left secondary" {
          }
          frame "Left primary" {
          }
        }
        n168 = call "PXI-StopDAQ.vi"("error in (no error)"=w394) -> ("error out"=w388:errorcluster)  [unwired: 6 in]
        n169 = case shown="False" w379 {
          tunnel: w399 -> [w432 _]
          tunnel: w398 -> [w431 _]
          tunnel: w397 -> [w430 _]
          tunnel: w396 -> [w429 _]
          tunnel: w389 -> [w428 _]
          tunnel: w388 -> [w427 w433]
          tunnel: w387 -> [w409 _]
          tunnel: w386 -> [w425 _]
          tunnel: w381 -> [w424 _]
          tunnel: w380 -> [w423 _]
          tunnel: [w422 w433] -> w373
          tunnel: [w421 _] -> w374
          tunnel: w376 -> [w420 _]
          tunnel: w369 -> [w408 _]
          frame False {
            n170 = call "CIE-Compute ASTF.vi"("Mag"=w432, "Stimulus"=w429, "Force no smoothing?"=w424, "Phase"=w431, "df (Hz)"=w430, "Probe Mic Gain (dB)"=w420, "error in (no error)"=w427, "Attenuation (dB)"=w423, "Probe Tube Path"=w428) -> ("Smooth Params"=w426:T8, "ASTF Mag"=w411:dbl[], "ASTF Phase"=w412:dbl[], "Frequency"=w415:dbl[], "Unsmoothed Mag"=w416:dbl[], "error out"=w419:errorcluster)  [unwired: 1 in]
            n171 = call "ACal-Remove Uncalibrated Frequencies.vi"("ASTF Mag in"=w411, "Cal Spec Out"=w409, "ASTF Phase in"=w412, "Frequency in"=w415, "Unsmoothed Mag in"=w416, "error in (no error)"=w419, "Weighted"=w408) -> ("ASTF Mag out"=w410:dbl[], "ASTF Phase out"=w413:dbl[], "Frequency out"=w414:dbl[], "Unsmoothed Mag out"=w417:dbl[], "error out"=w418:errorcluster)  [unwired: 4 in]
            n172 = call "CAL-Save Data V2.vi"("Mag"=w410, "Smooth Params"=w426, "Cal Stimulus"=w409, "Phase"=w413, "Frequency"=w414, "Unsmoothed Mag"=w417, "error in (no error)"=w418, "path"=w425, "Probe Tube File"=w428) -> ("new file path"=w421:path, "error out"=w422:errorcluster)  [unwired: 5 in]
          }
          frame True {
          }
        }
        n173 = Bundle("new file path"=w374, "error out"=w373) -> (w372:T9)  [unwired: 1 in]
        n174 = property on="result" class="Clust (strict)"("Val(Sgnl)"=w372) -> ()  [unwired: 2 in, 2 out]
      }
      frame Error {
      }
    }
  }
